vi "Open Cursor Digitizer.vi"(8 "error in (no error)":errorcluster, 11 "Spectrum Recorder in":refnum<class "Spectrum Recorder.lvclass">) -> (0 "error out":errorcluster, 3 "Spectrum Recorder out":refnum<class "Spectrum Recorder.lvclass">)   [LabVIEW 2016, in "Spectrum Recorder.lvclass"]
uses:
  Spectrum Recorder.lvclass
  Spectrum Recorder.lvclass/Spectrum Recorder.ctl
  <vilib>/ActorFramework/Message Enqueuer/Message Enqueuer.lvclass/Message Enqueuer.ctl
  <vilib>/ActorFramework/Message Enqueuer/Enqueue.vi
  Measure_core/Template Module Messages/Open Front Panel Msg/Open Front Panel Msg.lvclass
  C:/Program Files/National Instruments/LabVIEW 2016/vi.lib/ActorFramework/Message/Message.lvclass
  <vilib>/ActorFramework/Message Priority Queue/Priority Enqueue.vi
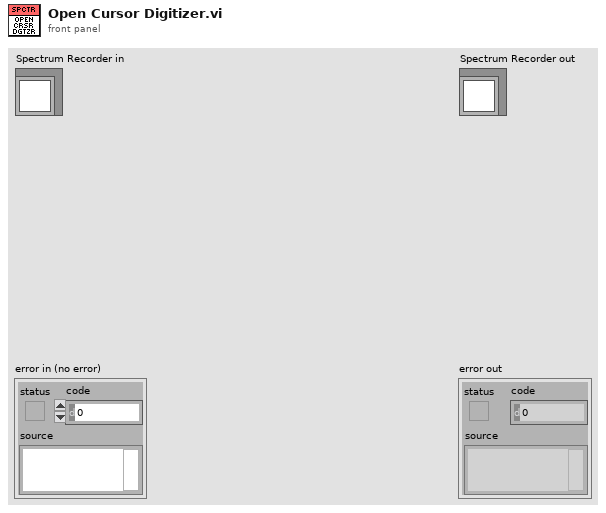
[diagram p1: front panel]
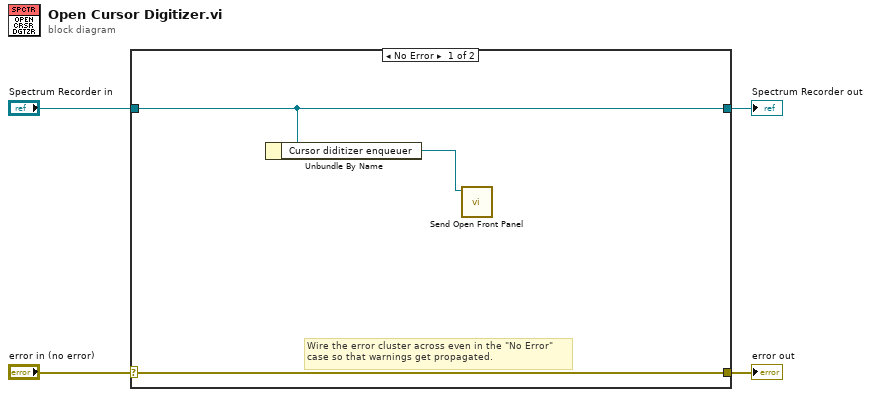
[diagram p0: block diagram]
diagram:
  n1 = case shown="No Error" "error in (no error)" {
    selector: "error in (no error)" -> [w7 w9]
    tunnel: [w7 w9] -> w3
    tunnel: [w6 w8] -> w1
    tunnel: "Spectrum Recorder in" -> [w6 w8]
    frame No Error {
      # "Wire the error cluster across even in the \"No Error\"\ncase so that warnings get propagated."
      n2 = Unbundle By Name(w6) -> ("Cursor diditizer enqueuer"=w5:refnum<class "Message Enqueuer.lvclass">)
      n3 = call "Send Open Front Panel.vi"("Message Enqueuer"=w5) -> ()  [unwired: 9 in, 2 out]
    }
    frame Error {
    }
  }
  "error out" <- w3
  "Spectrum Recorder out" <- w1
